vi "Set_Tunnel_Speed.vi"(3 "Mode":T1, 4 "Rig Name (default Empty)":string, 5 "Tunnel Velocity m/s":dbl min=0.0 max=50.0 format="%#.3f") -> (0 "Error String":string, 2 "Max allowable Tunnel Velocity":dbl)   [LabVIEW 2022 SP3]
doc: "This is an example of using features of the VI Server as a client. It shows how you might browse from one or more applications that may be exporting data from one or more data stations. \n\nThe example shows how to query a server for its list of exported VIs, how to get references to the VIs, and how call them with the Call By Reference function."
uses:
  Sub VIs/ADAM Controls/Tunnel_speed_mode.ctl
  Sub VIs/ADAM Controls/Channel_State.ctl
  Anemometry/Anemometry Sub Vis/File/Setup_Filetype.ctl
  Sub VIs/ADAM Controls/Update_scan_value.ctl
  Anemometry/Anemometry Sub Vis/Controls/Global_mode.ctl
  Sub VIs/ADAM Controls/Ch_description_ADAM.ctl
  Sub VIs/ADAM Controls/Module_type_ADAM.ctl
  Sub VIs/ADAM Controls/Function_ADAM.ctl
  Sub VIs/ADAM Controls/Calib_type_ADAM.ctl
  Sub VIs/ADAM Controls/Address.ctl
  Anemometry/Anemometry Sub Vis/Globals/Preference_global.vi
  Anemometry/Anemometry Sub Vis/Globals/Constants_global.vi
  <vilib>/Analysis/NI_AALPro.lvlib
panel:
  out "Motor Enable On?":bool
  out "i count":i32
  out "Settling Time (s)":dbl
  in  "Set EnFlo Tun Speed":refnum<vi>
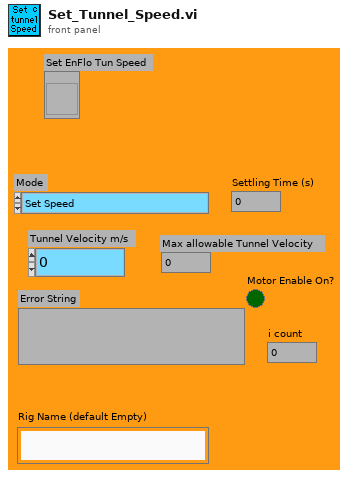
[diagram p1: front panel]
types:
  T1 = typedef "Tunnel_speed_mode.ctl" = enum16{"Set Speed", "Set Speed then wait", "Is tunnel speed allowable?"}
  T2 = typedef "Channel_State.ctl" = enum16{"On", "Off", "Always On", "Always Off"}
  T3 = enum16{"On", "Off", "Always On", "Always Off", "Delete"}
  T4 = typedef "Setup_Filetype.ctl" = enum16{"Measurement Setups", "Calibration Setups", "General", "Results File Plotter Setups", "Speed Calib Tweaks"}
  T5 = typedef "Calib_type_ADAM.ctl" = string
  T6 = typedef "Module_type_ADAM.ctl" = string
  T7 = typedef "Ch_description_ADAM.ctl" = cluster{"Ch Name":string, "Type":T6, "Function":T8, "Ch State":T2, "Calibration type":T5, "A":dbl, "B":dbl, "C":dbl, "D":dbl, "Comments":string, "Address":T9, "String":string, "Duty":u16}
  T8 = typedef "Function_ADAM.ctl" = enum16{"Analogue Input", "Digital Input", "Event counter", "Event rate", "Analogue Output", "Digital Output", "Relay Output"}
  T9 = typedef "Address.ctl" = cluster{"Main":i32, "Ch.":i32, "Sub":i32, "Port Name":string}
  T10 = typedef "Global_mode.ctl" = enum16{"Read Global", "Load Global From File", "Write Global to File"}
  T11 = typedef "Update_scan_value.ctl" = cluster{"Channel Name":string, "New Value":dbl, "!Auto_Off":bool}
  T12 = typedef "Server_Comms.ctl" = enum16{"Do Not Link To Server", "Server Link Healthy"}
  T13 = cluster{"second":i32, "minute":i32, "hour":i32, "day of month":i32, "month":i32, "year":i32, "day of week":i32, "day of year":i32, "is DST":i32}
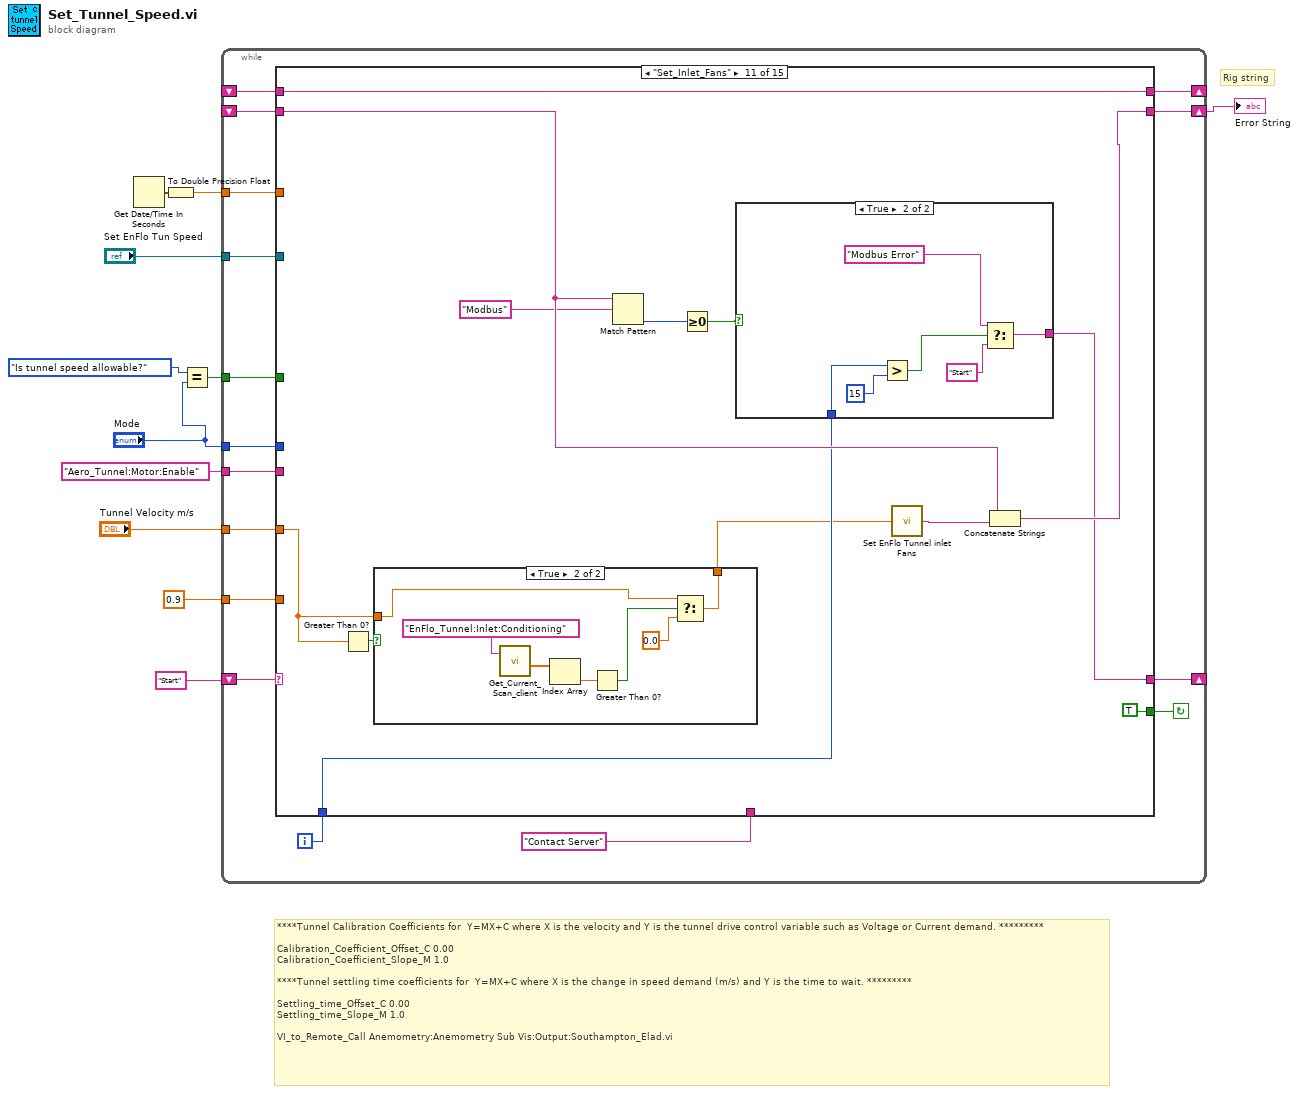
[diagram p0: block diagram]
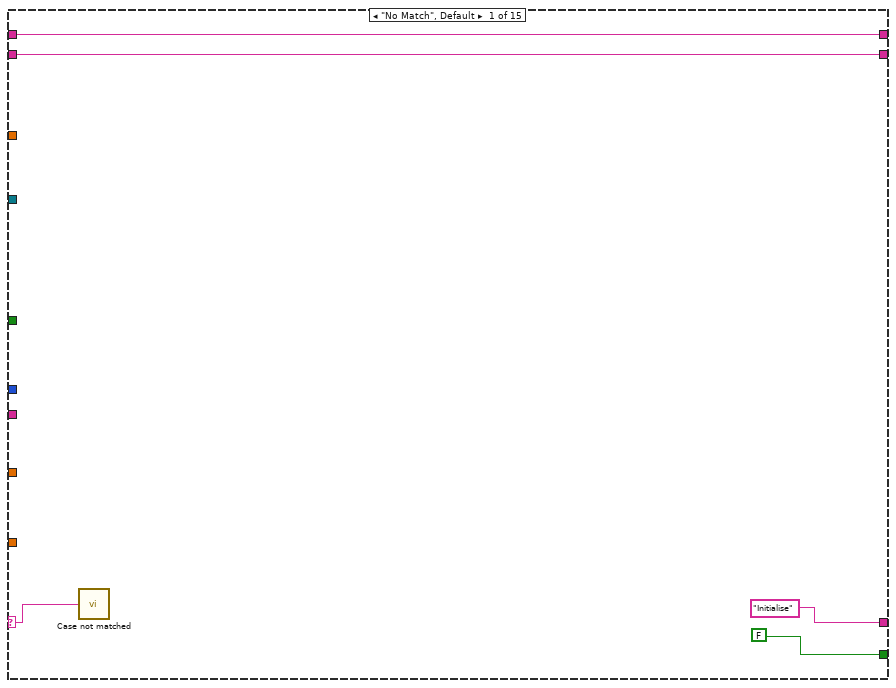
[diagram p2: hidden frame]
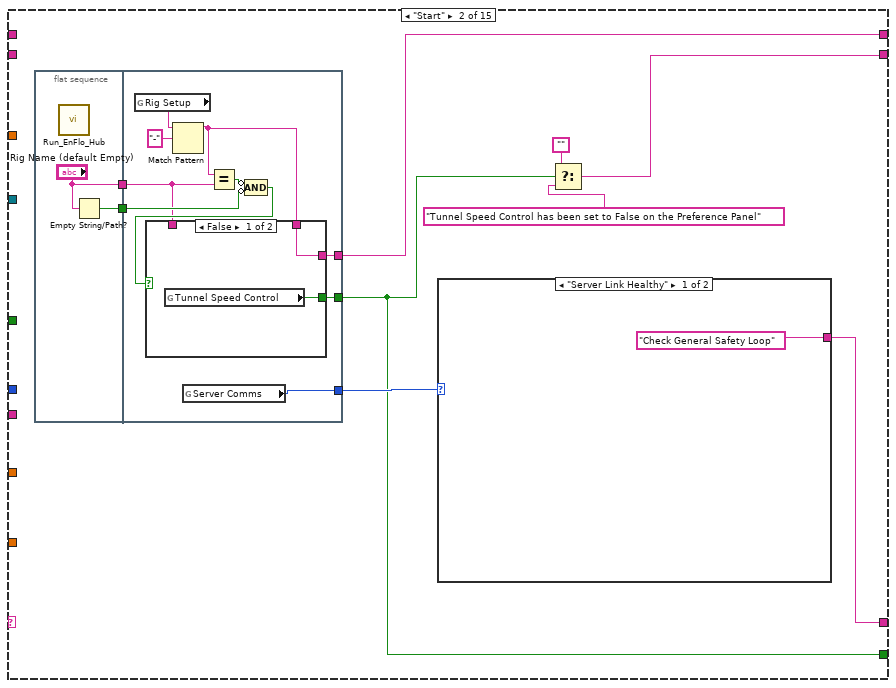
[diagram p3: hidden frame]
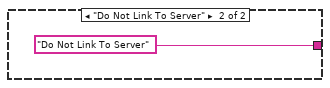
[diagram p4: hidden frame]
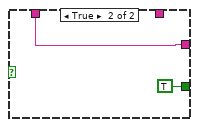
[diagram p5: hidden frame]
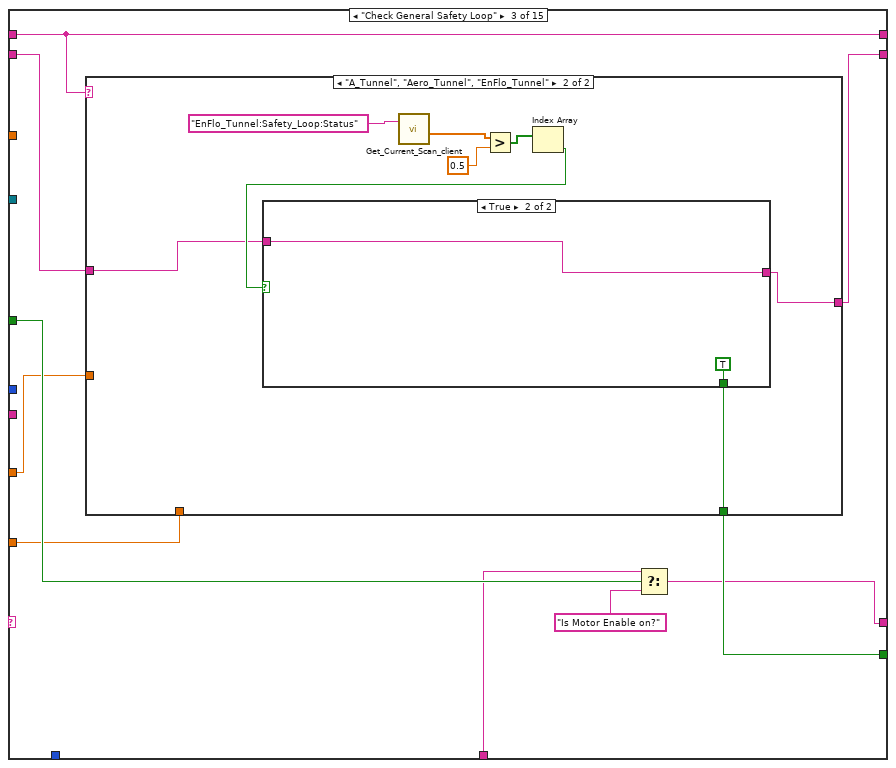
[diagram p6: hidden frame]
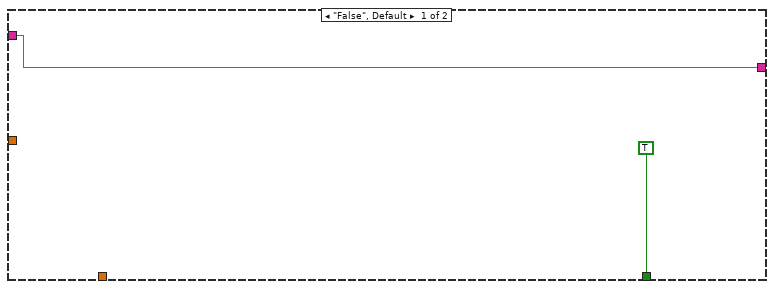
[diagram p7: hidden frame]
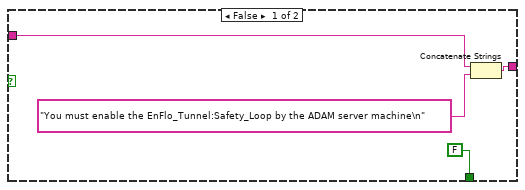
[diagram p8: hidden frame]
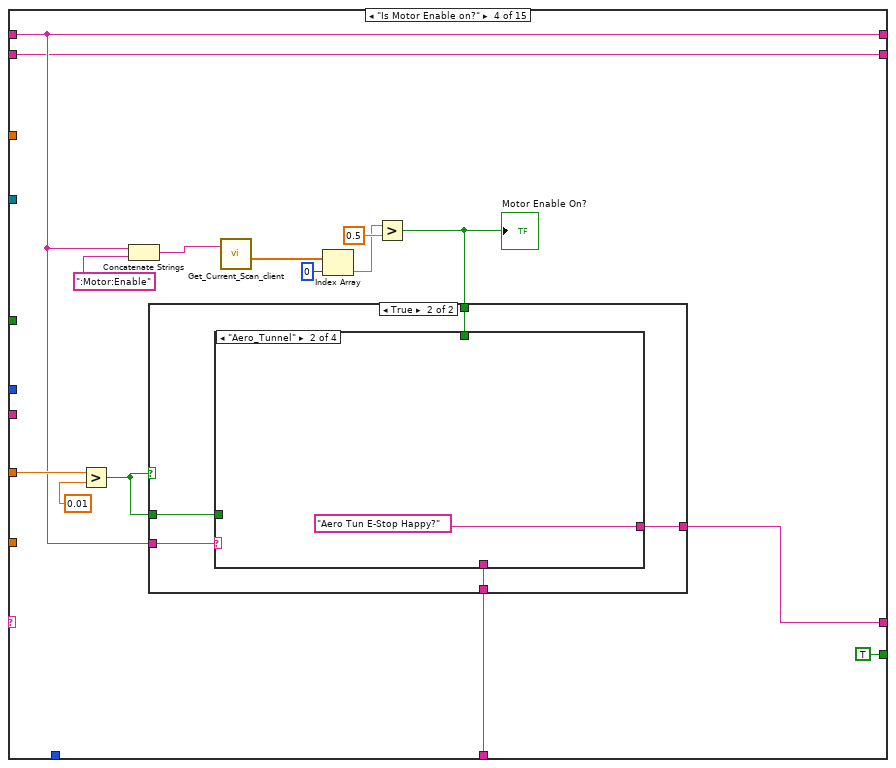
[diagram p9: hidden frame]
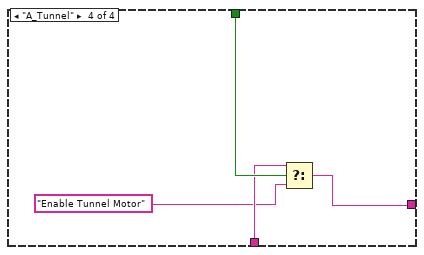
[diagram p13: hidden frame]
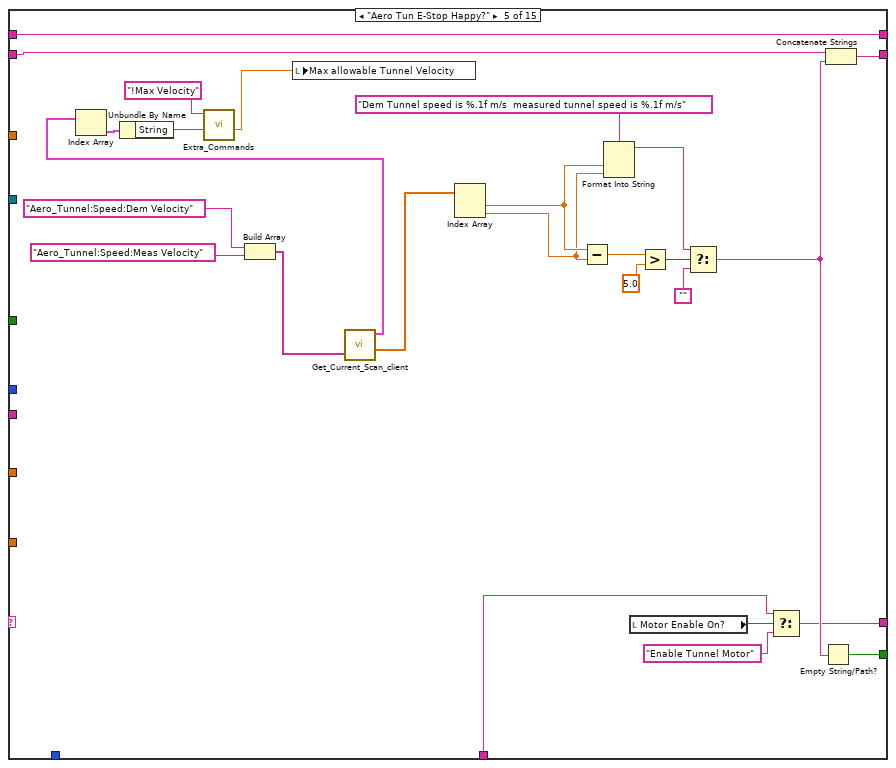
[diagram p14: hidden frame]
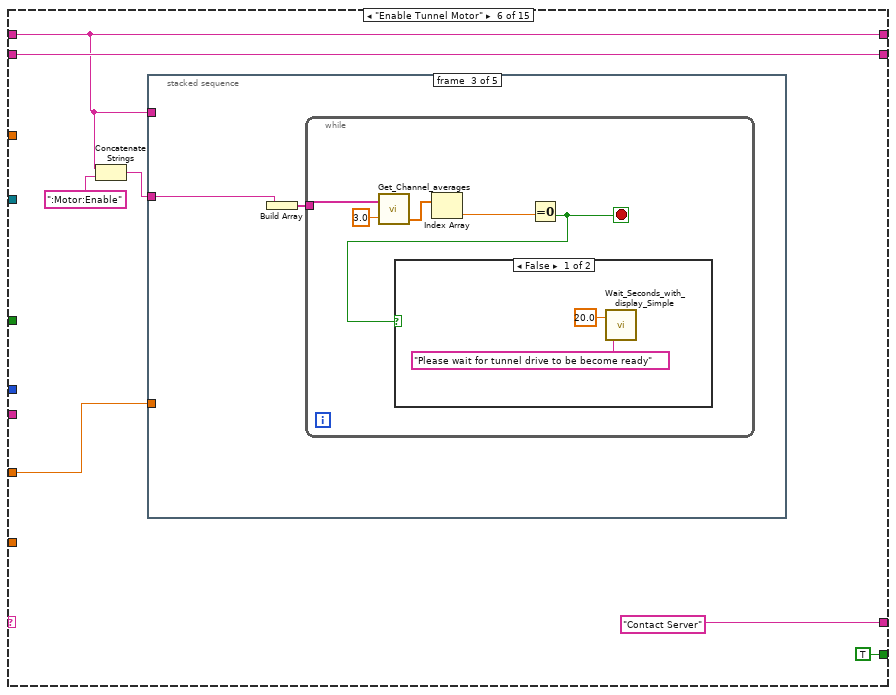
[diagram p15: hidden frame]
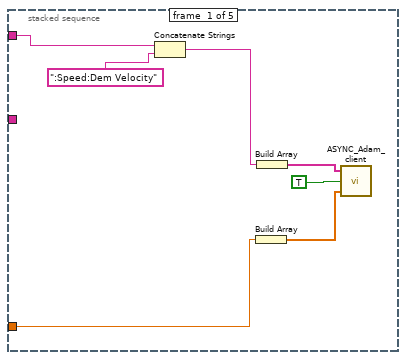
[diagram p16: hidden frame]
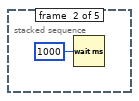
[diagram p17: hidden frame]
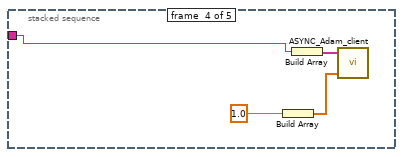
[diagram p19: hidden frame]
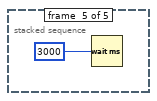
[diagram p20: hidden frame]
diagram:
  # "Rig string"
  # "****Tunnel Calibration Coefficients for  Y=MX+C where X is the velocity and Y is the tunnel drive control variable such as Voltage or Current demand. *********\n\nCalibration_Coefficient_Offset_C\t0.00\nCalibration_Coefficient_Slope_M\t1.0\n\n****Tunnel settling time coefficients for  Y=MX+C where X is the change in speed demand (m/s) and Y is the time to wait. *********\n\nSettling_time_Offset_C\t0.00\nSettling_time_Slope_M\t1.0\n\nVI_to_Remote_Call\tAnemometry:Anemometry Sub Vis:Output:Southampton_Elad.vi"
  n1 = Get Date/Time In Seconds() -> (seconds since 1Jan1904=w7:timestamp)
  n2 = To Double Precision Float(number=w7) -> (double precision float=w6:dbl)
  n3 = Equal?(x=Tunnel_speed_mode."Is tunnel speed allowable?" ("Mode"), y="Mode") -> (x = y?=w2:bool)
  n4 = while {
    shift-left: "Start" -> [w26]
    shift-right: [w27] -> _
    shift-right: [w25] -> w10
    shift-left: _ -> [w24]
    tunnel: "Mode" -> [w23]
    tunnel: "Tunnel Velocity m/s" -> [w22]
    shift-right: [w21] -> _
    shift-left: _ -> [w20]
    tunnel: "Set EnFlo Tun Speed" -> [w18]
    tunnel: w6 -> [w17]
    tunnel: "Aero_Tunnel:Motor:Enable" -> [w16]
    tunnel: 0.9 ("y") -> [w15]
    tunnel: w2 -> [w14]
    i -> [w13]
    stop <- w19 continue-if-true
    n5 = case shown="\"Set_Inlet_Fans\"" w26 {
      selector: w26 -> [w28 _ _ _ _ _ _ _ _ _ _ _ _ _ _]
      tunnel: [FALSE w40 w69 TRUE ("Tunnel Speed Control") w126 TRUE ("Tunnel Speed Control") w173 TRUE ("Tunnel Speed Control") w240 w357 TRUE ("Tunnel Speed Control") w427 w475 FALSE ("Tunnel Speed Control") FALSE] -> w19
      tunnel: ["Initialise" w36 w62 w92 w114 "Contact Server" ("f") w169 "Contact Server" ("f") w239 "Aero Tunnel Steady?" ("f") w401 w426 "Start" "End" ("f") "End"] -> w27
      tunnel: [w30 w38 w67 w89 w132 w146 w187 w215 w235 w381 w406 w430 w478 w499 w505] -> w25
      tunnel: w24 -> [w30 _ w68 w89 w133 w146 w189 w215 w236 w381 w405 w430 w478 w499 w503]
      tunnel: w23 -> [_ _ _ _ _ _ w186 _ w238 _ _ _ _ w492 w507]
      tunnel: w22 -> [_ _ w61 w94 _ w143 _ w222 w233 w360 w397 _ _ _ w506]
      tunnel: [w29 w35 w66 w93 w139 w140 w192 w211 w241 w382 w409 w431 w479 w500 w504] -> w21
      tunnel: w20 -> [w29 _ w66 w93 w139 w140 w192 w211 w241 w382 w409 w431 w479 w500 w504]
      tunnel: w18 -> [_ _ _ _ _ _ _ _ w242 _ _ _ _ _ _]
      tunnel: w17 -> [_ _ _ _ _ _ _ _ w234 _ _ _ _ _ _]
      tunnel: w16 -> [_ _ _ _ _ _ _ _ _ w344 _ _ _ _ _]
      tunnel: w15 -> [_ _ w60 _ _ _ _ _ w232 _ _ _ _ _ _]
      tunnel: w14 -> [_ _ w65 _ _ _ _ w214 w231 _ _ _ _ _ _]
      tunnel: w13 -> [_ _ _ _ _ _ _ _ _ w362 w400 w429 w477 _ _]
      tunnel: "Contact Server" ("f") -> [_ _ w64 w86 w115 _ _ _ _ _ _ _ _ _ _]
      frame "No Match", Default {
        n6 = call "Case not matched.vi"("Case Name not Matched"=w28) -> ()
      }
      frame "Start" {
        n7 = flat-sequence {
          tunnel: ["Rig Name (default Empty)"] -> w34
          tunnel: [w44] -> w33
          tunnel: [w55] -> w41
          tunnel: [w49] -> w40
          tunnel: [w48] -> w35
          tunnel: w34 -> [w46]
          tunnel: w33 -> [w51]
          frame #0 {
            n8 = call "Run_EnFlo_Hub.vi"() -> ()  [unwired: 1 in, 7 out]
            n9 = Empty String/Path?(string/path="Rig Name (default Empty)") -> (empty?=w44:bool)
          }
          frame #1 {
            n10 = global read "Preference_global.vi" "Rig Setup"() -> (w54:string)
            n11 = Match Pattern(string=w54, regular expression="-") -> (before substring=w47:string)  [unwired: 4 out]
            n12 = global read "Preference_global.vi" "Server Comms"() -> (w55:T12)
            n13 = Equal?(x=w47, y=w46) -> (x = y?=w52:bool)
            n14 = Compound Arithmetic op=AND(invert w52, invert w51) -> (w50:bool)
            n15 = case shown="False" w50 {
              tunnel: [w57 TRUE ("Tunnel Speed Control")] -> w49
              tunnel: [w56 w58] -> w48
              tunnel: w47 -> [w56 _]
              tunnel: w46 -> [_ w58]
              frame False {
                n16 = global read "Preference_global.vi" "Tunnel Speed Control"() -> (w57:bool)
              }
              frame True {
              }
            }
          }
        }
        n17 = case shown="\"Server Link Healthy\"" w41 {
          tunnel: ["Check General Safety Loop" "Do Not Link To Server"] -> w36
          frame "Server Link Healthy" {
          }
          frame "Do Not Link To Server" {
          }
        }
        n18 = Select(t="", s=w40, f="Tunnel Speed Control has been set to False on the Preference Panel" ("Error String")) -> (s? t:f=w38:string)
      }
      frame "Check General Safety Loop" {
        n19 = case shown="\"A_Tunnel\", \"Aero_Tunnel\", \"EnFlo_Tunnel\"" w66 {
          tunnel: w68 -> [w70 w74]
          tunnel: [w70 w73] -> w67
          tunnel: [TRUE ("Tunnel Speed Control") w72] -> w69
          tunnel: w61 -> [_ _]
          tunnel: w60 -> [_ _]
          frame "False", Default {
          }
          frame "A_Tunnel", "Aero_Tunnel", "EnFlo_Tunnel" {
            n20 = call "Get_Current_Scan_client.vi"("singleChannel"="EnFlo_Tunnel:Safety_Loop:Status") -> ("Numerical Values"=w77:dbl[])  [unwired: 1 in, 3 out]
            n21 = Greater?(x=w77, y=0.5) -> (0:w78:bool[])
            n22 = Index Array(array=w78) -> (element=w75:bool)  [unwired: 1 in]
            n23 = case shown="True" w75 {
              tunnel: [w83 w84] -> w73
              tunnel: w74 -> [w81 w84]
              tunnel: [FALSE ("Tunnel Speed Control") TRUE ("Tunnel Speed Control")] -> w72
              frame False {
                n24 = Concatenate Strings(w81, "You must enable the EnFlo_Tunnel:Safety_Loop by the ADAM server machine\n") -> (w83:string)
              }
              frame True {
              }
            }
          }
        }
        n25 = Select(t=w64, s=w65, f="Is Motor Enable on?") -> (s? t:f=w62:string)
      }
      frame "Is Motor Enable on?" {
        n26 = Greater?(x=w94, y=0.01) -> (0:w88:bool)
        n27 = Concatenate Strings(w93, ":Motor:Enable" ("string")) -> (w91:string)
        n28 = call "Get_Current_Scan_client.vi"("singleChannel"=w91) -> ("Numerical Values"=w96:dbl[])  [unwired: 1 in, 3 out]
        n29 = Index Array(array=w96, index=0) -> (element=w98:dbl)
        n30 = Greater?(x=w98, y=0.5) -> (0:w90:bool)
        "Motor Enable On?" <- w90
        n31 = case shown="True" w88 {
          tunnel: w93 -> [_ w106]
          tunnel: w86 -> [w101 w105]
          tunnel: [w101 w104] -> w92
          tunnel: w90 -> [_ w103]
          tunnel: w88 -> [_ w102]
          frame False {
          }
          frame True {
            n32 = case shown="\"Aero_Tunnel\"" w106 {
              selector: w106 -> [_ _ w109 _]
              tunnel: [w107 "Aero Tun E-Stop Happy?" ("f") w109 w110] -> w104
              tunnel: w105 -> [w107 _ _ w112]
              tunnel: w103 -> [_ _ _ w113]
              tunnel: w102 -> [_ _ _ _]
              frame Default {
              }
              frame "Aero_Tunnel" {
              }
              frame "EnFlo_Tunnel" {
              }
              frame "A_Tunnel" {
                n33 = Select(t=w112, s=w113, f="Enable Tunnel Motor") -> (s? t:f=w110:string)
              }
            }
          }
        }
      }
      frame "Aero Tun E-Stop Happy?" {
        n34 = Build Array("Aero_Tunnel:Speed:Dem Velocity", "Aero_Tunnel:Speed:Meas Velocity") -> (w136:string[])
        n35 = call "Get_Current_Scan_client.vi"("multipleChannels"=w136) -> ("Ch Description Array"=w123:T7[], "Numerical Values"=w119:dbl[])  [unwired: 1 in, 2 out]
        n36 = Index Array(array=w123) -> (element=w122:T7)  [unwired: 1 in]
        n37 = Unbundle By Name(w122) -> ("String"=w124:string)
        n38 = call "Extra_Commands.vi"("String to Search"=w124, "Command"="!Max Velocity") -> ("Numeric Value"=w121:dbl)  [unwired: 1 in, 4 out]
        n39 = local write "Max allowable Tunnel Velocity"(w121) -> ()
        n40 = Index Array(array=w119) -> (element #1=w131:dbl, element #2=w118:dbl)  [unwired: 2 in]
        n41 = Subtract(x=w131, y=w118) -> (x-y=w135:dbl)
        n42 = Format Into String(format string="Dem Tunnel speed is %.1f m/s  measured tunnel speed is %.1f m/s", w131, w118) -> (resulting string=w129:string)  [unwired: 2 in, 1 out]
        n43 = local read "Motor Enable On?"() -> (w117:bool)
        n44 = Greater?(x=w135, y=5.0) -> (0:w128:bool)
        n45 = Select(t=w129, s=w128, f="") -> (s? t:f=w120:string)
        n46 = Select(t=w115, s=w117, f="Enable Tunnel Motor") -> (s? t:f=w114:string)
        n47 = Empty String/Path?(string/path=w120) -> (empty?=w126:bool)
        n48 = Concatenate Strings(w133, w120) -> (w132:string)
      }
      frame "Enable Tunnel Motor" {
        n49 = Concatenate Strings(w140, ":Motor:Enable" ("string")) -> (w141:string)
        n50 = stacked-sequence {
          tunnel: w141 -> [_ _ w156 w164 _]
          tunnel: w143 -> [w151 _ _ _ _]
          tunnel: w140 -> [w149 _ _ _ _]
          frame #0 {
            n51 = Concatenate Strings(w149, ":Speed:Dem Velocity" ("string")) -> (w147:string)
            n52 = Build Array(w151) -> (w150:dbl[])
            n53 = Build Array(w147) -> (w153:string[])
            n54 = call "ASYNC_Adam_client.vi"("Values"=w150, "Check Value is in the scan table?"=TRUE, "Channel Names"=w153) -> ()  [unwired: 2 out]
          }
          frame #1 {
            n55 = Wait (ms)(milliseconds to wait=u32 1000) -> ()  [unwired: 1 out]
          }
          frame #2 {
            n56 = Build Array(w156) -> (w155:string[])
            n57 = while {
              tunnel: w155 -> [w161]
              stop <- w157 stop-if-true
              n58 = call "Get_Channel_averages.vi"("Desired Ch Names"=w161, "Averaging time (mins)"=3.0) -> ("number"=w159:dbl[])  [unwired: 1 in, 2 out]
              n59 = Index Array(array=w159) -> (element=w158:dbl)  [unwired: 1 in]
              n60 = Equal To 0?(x=w158) -> (x = 0?=w157:bool)
              n61 = case shown="False" w157 {
                frame False {
                  n62 = call "Wait_Seconds_with_display_Simple.vi"("Message"="Please wait for tunnel drive to be become ready", "Seconds to wait"=20.0) -> ()  [unwired: 1 in, 1 out]
                }
                frame True {
                }
              }
            }
          }
          frame #3 {
            n63 = Build Array(1.0 ("y")) -> (w166:dbl[])
            n64 = Build Array(w164) -> (w165:string[])
            n65 = call "ASYNC_Adam_client.vi"("Values"=w166, "Channel Names"=w165) -> ()  [unwired: 1 in, 2 out]
          }
          frame #4 {
            n66 = Wait (ms)(milliseconds to wait=u32 3000 ("millisecond timer value")) -> ()  [unwired: 1 out]
          }
        }
      }
      frame "EnFlo_Tunnel" {
        w175 = "EnFlo_Tunnel:Drive:In Standby"
        w182 = "EnFlo_Tunnel:Bus Bar + Heaters:Enable"
        n67 = Build Array(w182, w175, "EnFlo_Tunnel:Emergency_Stop:Happy") -> (w190:string[])
        n68 = call "Get_Current_Scan_client.vi"("multipleChannels"=w190) -> ("Ch Description Array"=w181:T7[], "Numerical Values"=w185:dbl[])  [unwired: 1 in, 2 out]
        n69 = Greater?(x=w185, y=0.5) -> (0:w184:bool[])
        n70 = Index Array(array=w184) -> (element #1=w183:bool, element #3=w173:bool)  [unwired: 3 in, 1 out]
        n71 = case shown="True" w173 {
          tunnel: w182 -> [_ w200]
          tunnel: ["The EnFlo_Tunnel Emergency Stop button has been pressed. You need to reset it before running." w199] -> w188
          tunnel: w186 -> [_ w198]
          tunnel: w183 -> [_ w197]
          frame False {
          }
          frame True {
            n72 = case shown="False" w197 {
              tunnel: w200 -> [w203 _]
              tunnel: ["" ""] -> w199
              tunnel: w198 -> [w201 _]
              frame False {
                n73 = case shown="Default" w201 {
                  tunnel: w203 -> [_ w207]
                  frame "Is tunnel speed allowable?" {
                  }
                  frame Default {
                    n74 = Build Array(w207, "EnFlo_Tunnel:Shutting:Down") -> (w206:string[])
                    n75 = Build Array(1.0 ("element"), 0.0 ("element")) -> (w209:dbl[])
                    n76 = call "ASYNC_Adam_client.vi"("Values"=w209, "Channel Names"=w206) -> ()  [unwired: 1 in, 2 out]
                  }
                }
              }
              frame True {
              }
            }
          }
        }
        n77 = Index Array(array=w181, index=1) -> (element=w179:T7)
        n78 = Unbundle By Name(w179) -> ("Ch State"=w178:T2)
        n79 = local read "Motor Enable On?"() -> (w172:bool)
        n80 = Equal?(x=w178, y=Channel_State."Off") -> (x = y?=w176:bool)
        n81 = Concatenate Strings(w189, w188) -> (w187:string)
        n82 = case shown="True" w176 {
          tunnel: w175 -> [_ w195]
          frame False {
          }
          frame True {
            n83 = Build Array(w195) -> (w194:string[])
            n84 = call "Cntrl_Ch_Status_low.vi"("Mode"=T3."On", "Channel names"=w194) -> ()  [unwired: 1 out]
          }
        }
        n85 = Select(t="Contact Server" ("f"), s=w172, f="Enable EnFlo Tunnel Motor") -> (s? t:f=w169:string)
      }
      frame "Enable EnFlo Tunnel Motor" {
        n86 = Greater?(x=w222, y=0.15) -> (0:w220:bool)
        n87 = Concatenate Strings(w211, ":Motor:Enable" ("string")) -> (w212:string)
        n88 = Build Array(w212) -> (w217:string[])
        n89 = Compound Arithmetic op=AND(w220, invert w214) -> (w218:bool)
        n90 = case shown="True" w218 {
          tunnel: w217 -> [_ w223]
          frame False {
          }
          frame True {
            n91 = stacked-sequence {
              tunnel: w223 -> [w227 _]
              frame #0 {
                n92 = Build Array(1.0 ("y")) -> (w229:dbl[])
                n93 = Build Array("EnFlo_Tunnel:Drive:In Standby") -> (w226:string[])
                n94 = call "ASYNC_Adam_client.vi"("Values"=w229, "Channel Names"=w227) -> ()  [unwired: 1 in, 2 out]
                n95 = call "Cntrl_Ch_Status_low.vi"("Mode"=T3."On", "Channel names"=w226) -> ()  [unwired: 1 out]
              }
              frame #1 {
                n96 = Wait (ms)(milliseconds to wait=u32 3000 ("millisecond timer value")) -> ()  [unwired: 1 out]
              }
            }
          }
        }
      }
      frame "Contact Server" {
        n97 = while {
          tunnel: w238 -> [w278]
          tunnel: w233 -> [w279]
          shift-left: _ -> [w275]
          shift-right: [w282] -> _
          tunnel: [w277] -> w237
          tunnel: w241 -> [w276]
          tunnel: w242 -> [w274]
          tunnel: w234 -> [w273]
          i -> [w281]
          stop <- w280 continue-if-true
          n98 = stacked-sequence {
            seq-local: [_ w291 _ _] -> [_ _ w299 _]
            seq-local: [_ w290 _ _] -> [_ _ w297 _]
            seq-local: [_ _ w293 _] -> [_ _ _ w325]
            tunnel: w275 -> [_ w292 _ _]
            tunnel: [_ _ w300 _] -> w282
            tunnel: w281 -> [_ _ _ w326]
            tunnel: [_ _ _ w324] -> w280
            tunnel: w279 -> [_ w288 _ _]
            tunnel: w278 -> [_ w284 _ _]
            tunnel: [_ w286 _ _] -> w277
            tunnel: w276 -> [_ w285 _ _]
            tunnel: w274 -> [_ _ w296 _]
            tunnel: w273 -> [_ _ w294 _]
            frame #0 {
            }
            frame #1 {
              n99 = call "Full_Client_Name.vi"() -> ("Client Name"=w289:string)
              n100 = call-by-ref "?"(reference=w292, "Tunnel Velocity m/s"=w288, "Rig Name"=w285, "Mode"=w284, "Client Name"=w289) -> (reference out=w291:refnum<vi>, error out=w290:errorcluster, "Error String"=w286:string, "Settling Time (s)"=→"Settling Time (s)":dbl, "Max allowable Tunnel Velocity"=→"Max allowable Tunnel Velocity":dbl)  [unwired: 1 in, 1 out]
            }
            frame #2 {
              n101 = Unbundle By Name(w297) -> ("status"=w298:bool)
              n102 = case shown="False" w298 {
                selector: w298 -> [w301 _]
                tunnel: [w302 w309] -> w300
                tunnel: w299 -> [w302 _]
                tunnel: [w303 w308] -> w295
                tunnel: w297 -> [w303 _]
                tunnel: w296 -> [_ w307]
                tunnel: [w301 w305] -> w293
                frame False {
                }
                frame True {
                  n103 = call "Start_Client_Coms.vi"("VI name to run on server"="Set_Tunnel_Speed_server.vi") -> ("LabVIEW application reference"=w311:refnum<vi>, "Checked VI name"=w312:path, "Local Call"=w310:bool, "Error cluster"=w304:errorcluster)  [unwired: 1 in]
                  n104 = case shown="False" w310 {
                    tunnel: [w318 w323] -> w309
                    tunnel: w307 -> [w316 w322]
                    tunnel: w312 -> [w315 w321]
                    tunnel: w311 -> [w314 _]
                    tunnel: [w317 w320] -> w308
                    frame False {
                      n105 = Strip Path(path=w315) -> (name=w319:string)  [unwired: 1 out]
                      n106 = Open VI Reference(type specifier VI Refnum (for type only)=w316, application reference (local)=w314, vi path=w319) -> (vi reference=w318:refnum<vi>, error out=w317:errorcluster)  [unwired: 1 in, 2 out]
                    }
                    frame True {
                      n107 = Open VI Reference(type specifier VI Refnum (for type only)=w322, vi path=w321) -> (vi reference=w323:refnum<vi>, error out=w320:errorcluster)  [unwired: 1 in, 3 out]
                    }
                  }
                  n108 = Unbundle By Name(w304) -> ("status"=w306:bool)
                  n109 = Not(x=w306) -> (.not. x?=w305:bool)
                }
              }
              n110 = call "Delay Error Message.vi"("error in (no error)"=w295, "Seconds since 1904"=w294) -> ()  [unwired: 2 in]
            }
            frame #3 {
              n111 = Less?(x=w326, y=30) -> (x < y?=w328:bool)
              n112 = And(x=w328, y=w325) -> (x .and. y?=w324:bool)
            }
          }
        }
        n113 = case shown="\"EnFlo_Tunnel\"" w241 {
          tunnel: [TRUE w248 w268] -> w240
          tunnel: ["Tunnel Speed Settling" ("f") "Aero Tunnel Steady?" ("f") "Set_Inlet_Fans" ("f")] -> w239
          tunnel: w238 -> [_ w249 w270]
          tunnel: w233 -> [_ w247 _]
          tunnel: w232 -> [_ w246 _]
          tunnel: w231 -> [_ w245 _]
          frame "No Match", Default {
          }
          frame "Aero_Tunnel" {
            n114 = case shown="False" w245 {
              tunnel: w247 -> [w260 _]
              tunnel: w246 -> [w259 _]
              frame False {
                w252 = "Aero_Tunnel:Motor:Engaged"
                n115 = Greater?(x=w260, y=w259) -> (0:w253:bool)
                n116 = call "Get_Current_Scan_client.vi"("singleChannel"=w252) -> ("Numerical Values"=w258:dbl[])  [unwired: 1 in, 3 out]
                n117 = Index Array(array=w258) -> (element=w257:dbl)  [unwired: 1 in]
                n118 = Greater?(x=w257, y=0.5) -> (0:w255:bool)
                n119 = Equal?(x=w255, y=w253) -> (x = y?=w254:bool)
                n120 = case shown="False" w254 {
                  tunnel: w252 -> [w266 _]
                  tunnel: w253 -> [w264 _]
                  frame False {
                    n121 = Select(t=1.0, s=w264, f=0.0) -> (s? t:f=w261:dbl)
                    n122 = Build Array(w266) -> (w265:string[])
                    n123 = Build Array(w261) -> (w267:dbl[])
                    n124 = call "ASYNC_Adam_client.vi"("Values"=w267, "Channel Names"=w265) -> ()  [unwired: 1 in, 2 out]
                  }
                  frame True {
                  }
                }
              }
              frame True {
              }
            }
            n125 = Equal?(x=Tunnel_speed_mode."Set Speed then wait" ("Mode"), y=w249) -> (x = y?=w248:bool)
          }
          frame "EnFlo_Tunnel" {
            n126 = Equal?(x=Tunnel_speed_mode."Is tunnel speed allowable?" ("Mode"), y=w270) -> (x = y?=w269:bool)
            n127 = Not(x=w269) -> (.not. x?=w268:bool)
          }
        }
        n128 = Concatenate Strings(w236, w237) -> (w235:string)
      }
      frame "Aero Tunnel Steady?" {
        w351 = string[] ["Aero_Tunnel:Speed:Meas Velocity", "Aero_Tunnel:Speed:Dem Velocity"] ("ADAM Ch Names")
        n129 = Index Array(array=w351, index=1) -> (element=w349:string)
        n130 = Build Array(w349, w344) -> (w348:string[])
        n131 = call "Get_Ch_Time_Trace.vi"("Desired Ch Names"=w348, "History Length (mins)"=4.0) -> ("Output array"=w342:dbl[][])  [unwired: 2 out]
        n132 = Index Array(array=w342, index (row)=1) -> (element=w340:dbl[])  [unwired: 1 in]
        n133 = Equal To 0?(x=w340) -> (x = 0?=w341:bool[])
        n134 = Index Array(array=w342, index (row)=0) -> (element=w346:dbl[])  [unwired: 1 in]
        n135 = call "Get_Ch_Time_Trace.vi"("Desired Ch Names"=w351, "History Length (mins)"=0.3) -> ("Centre Times"=w335:dbl[], "Output array"=w377:dbl[][])  [unwired: 1 out]
        n136 = And Array Elements(Boolean array=w341) -> (logical AND=w338:bool)
        n137 = Equal To 0?(x=w346) -> (x = 0?=w345:bool[])
        n138 = And Array Elements(Boolean array=w345) -> (logical AND=w339:bool)
        n139 = Greater?(x=w360, y=4.0) -> (0:w358:bool)
        n140 = Less?(x=w362, y=18) -> (x < y?=w355:bool)
        n141 = Or(x=w339, y=w338) -> (x .or. y?=w337:bool)
        n142 = Index Array(array=w377, index (row)=0) -> (element=w336:dbl[])  [unwired: 1 in]
        n143 = Index Array(array=w377, index (row)=1) -> (element=w369:dbl[])  [unwired: 1 in]
        n144 = call "Mean_fr_NaN_data.vi"("Data"=w369) -> ("Mean value"=w368:dbl)  [unwired: 1 out]
        n145 = call <vilib>:"Linear Fit.vi"("Y"=w336, "X"=w335) -> ("Best Linear Fit"=w333:dbl[])  [unwired: 9 in, 4 out]
        n146 = Subtract(x=w368, y=w360) -> (x-y=w374:dbl)
        n147 = Array Size(array=w333) -> (size(s)=w332:i32)
        n148 = In Range and Coerce(upper limit=0.01, x=w374, lower limit=-0.01) -> (In Range?=w373:bool)  [unwired: 1 out]
        n149 = Decrement(x=w332) -> (x-1=w331:i32)
        n150 = Not A Number/Path/Refnum?(number/path/refnum=w368) -> (NaN/Path/Refnum?=w370:bool)
        n151 = Not A Number/Path/Refnum?(number/path/refnum=w336) -> (NaN/Path/Refnum?=w354:bool[])
        n152 = Not(x=w373) -> (.not. x?=w372:bool)
        n153 = And Array Elements(Boolean array=w354) -> (logical AND=w353:bool)
        n154 = Index Array(array=w333, index #1=0 ("index"), index #2=w331) -> (element #1=w330:dbl, element #2=w329:dbl)
        n155 = Subtract(x=w330, y=w329) -> (x-y=w365:dbl)
        n156 = In Range and Coerce(upper limit=0.2, x=w365, lower limit=-0.2) -> (In Range?=w364:bool)  [unwired: 1 out]
        n157 = Not(x=w364) -> (.not. x?=w363:bool)
        n158 = Or(x=w363, y=w372) -> (x .or. y?=w371:bool)
        n159 = Compound Arithmetic op=AND(invert w353, w371, invert w370) -> (w356:bool)
        n160 = case shown="True" w337 {
          tunnel: w358 -> [w387 _]
          tunnel: [w386 FALSE] -> w357
          tunnel: w356 -> [w385 _]
          tunnel: w355 -> [w384 _]
          frame False {
            n161 = case shown="False" w387 {
              tunnel: [w389 w393] -> w386
              tunnel: w385 -> [w390 w393]
              tunnel: w384 -> [w388 _]
              frame False {
                n162 = case shown="True" w390 {
                  selector: w390 -> [w391 _]
                  tunnel: [w391 w392] -> w389
                  tunnel: w388 -> [_ w392]
                  frame False {
                  }
                  frame True {
                  }
                }
              }
              frame True {
              }
            }
          }
          frame True {
          }
        }
        n163 = case shown="True" w357 {
          frame False {
          }
          frame True {
            n164 = call "Wait_Seconds_with_display.vi"("Message"="Tunnel speed settling", "Seconds to wait"=4.0) -> ()  [unwired: 2 out]
          }
        }
        "i count" <- w362
      }
      frame "Set_Inlet_Fans" {
        n165 = Greater Than 0?(x=w397) -> (x > 0?=w399:bool)
        n166 = case shown="True" w399 {
          tunnel: [w410 w411] -> w398
          tunnel: w397 -> [w410 w413]
          frame False {
          }
          frame True {
            n167 = call "Get_Current_Scan_client.vi"("singleChannel"="EnFlo_Tunnel:Inlet:Conditioning") -> ("Numerical Values"=w416:dbl[])  [unwired: 1 in, 3 out]
            n168 = Index Array(array=w416) -> (element=w415:dbl)  [unwired: 1 in]
            n169 = Greater Than 0?(x=w415) -> (x > 0?=w414:bool)
            n170 = Select(t=w413, s=w414, f=0.0) -> (s? t:f=w411:dbl)
          }
        }
        n171 = Match Pattern(string=w405, regular expression="Modbus") -> (offset past match=w403:i32)  [unwired: 1 in, 3 out]
        n172 = Greater Or Equal To 0?(x=w403) -> (x >= 0?=w402:bool)
        n173 = case shown="True" w402 {
          tunnel: ["Tunnel Speed Settling" ("f") w419] -> w401
          tunnel: w400 -> [_ w423]
          frame False {
          }
          frame True {
            n174 = Greater?(x=w423, y=15) -> (0:w422:bool)
            n175 = Select(t="Modbus Error", s=w422, f="Start") -> (s? t:f=w419:string)
          }
        }
        n176 = call "Set EnFlo Tunnel inlet Fans.vi"("Tunnel Velocity m/s"=w398) -> ("Error Message"=w407:string)
        n177 = Concatenate Strings(w405, w407) -> (w406:string)
      }
      frame "Modbus Error" {
        n178 = disable-structure shown="Enabled" {
          disable-tunnel: [w433 w468] -> w426
          disable-tunnel: "Reset EnFlo Tunnel Modbus" -> [w432 w468]
          frame Disabled {
            n179 = Get Date/Time In Seconds() -> (seconds since 1Jan1904=w439:timestamp)
            n180 = call <vilib>:"LV70TimeStampToDateRec.vi"("time stamp"=w439) -> ("date time rec"=w440:T13)
            n181 = Unbundle By Name(w440) -> ("hour"=w442:i32, "day of week"=w441:i32)
            n182 = In Range and Coerce(upper limit=16 ("lower limit"), x=w442, lower limit=8) -> (In Range?=w444:bool)  [unwired: 1 out]
            n183 = In Range and Coerce(upper limit=7, x=w441, lower limit=1) -> (In Range?=w443:bool)  [unwired: 1 out]
            n184 = And(x=w444, y=w443) -> (x .and. y?=w434:bool)
            n185 = case shown="True" w434 {
              tunnel: [w445 w447] -> w433
              tunnel: w432 -> [w445 w446]
              frame False {
              }
              frame True {
                n186 = stacked-sequence {
                  seq-local: [_ w451 _ _] -> [_ _ w455 _]
                  seq-local: [_ _ w454 _] -> [_ _ _ w463]
                  tunnel: [_ _ _ w461] -> w447
                  tunnel: w446 -> [_ _ _ w462]
                  frame #0 {
                    n187 = call "Email_With_Log.vi"("recipients"=string[] ["paulhayden28@gmail.com", "p.hayden@surrey.ac.uk"], "subject ([No Subject])"="Modbus Error", "message"="Please come and investigate") -> ()  [unwired: 1 in, 3 out]
                  }
                  frame #1 {
                    n188 = call "Wait_Seconds_with_display.vi"("Message"="Press Stop when Ready to make a Decision Regard the Modbus error", "Seconds to wait"=1800 ("y")) -> ("Stopped"=w451:bool)  [unwired: 1 out]
                  }
                  frame #2 {
                    n189 = case shown="True" w455 {
                      tunnel: [FALSE ("T button?") w457] -> w454
                      frame False {
                      }
                      frame True {
                        n190 = Two Button Dialog(message="Do you want to investigate the Modbus error?", 1:"No, Just do the usual Reset" ("F button name (\"Cancel\")"), 2:"Yes" ("T button name (\"OK\")")) -> (T button?=w457:bool)
                      }
                    }
                  }
                  frame #3 {
                    n191 = case shown="True" w463 {
                      tunnel: [w464 "Start"] -> w461
                      tunnel: w462 -> [w464 _]
                      frame False {
                      }
                      frame True {
                        n192 = call "Wait_Seconds_with_display.vi"("Message"="Press Stop when you want the code to try again", "Seconds to wait"=4000.0) -> ()  [unwired: 2 out]
                      }
                    }
                  }
                }
              }
            }
          }
          frame Enabled {
          }
        }
        n193 = Less?(x=w429, y=30) -> (x < y?=w427:bool)
      }
      frame "Reset EnFlo Tunnel Modbus" {
        w470 = "EnFlo_Tunnel:Modbus:Reset"
        n194 = Less?(x=w477, y=30) -> (x < y?=w475:bool)
        n195 = Build Array(w470) -> (w474:string[])
        n196 = stacked-sequence {
          tunnel: w474 -> [w483 _ w488 _]
          frame #0 {
            n197 = Build Array(1.0) -> (w481:dbl[])
            n198 = call "ASYNC_Adam_client.vi"("Values"=w481, "Channel Names"=w483) -> ()  [unwired: 1 in, 2 out]
          }
          frame #1 {
            n199 = call "Wait_Seconds_with_display.vi"("Message"="Resetting EnFlo_Tunnel Modbus", "Seconds to wait"=15.0) -> ()  [unwired: 1 in, 1 out]
          }
          frame #2 {
            n200 = Build Array(0.0) -> (w486:dbl[])
            n201 = call "ASYNC_Adam_client.vi"("Values"=w486, "Channel Names"=w488) -> ()  [unwired: 1 in, 2 out]
          }
          frame #3 {
            n202 = call "Wait_Seconds_with_display.vi"("Message"="Reconnecting EnFlo_Tunnel Modbus", "Seconds to wait"=15.0) -> ()  [unwired: 1 in, 1 out]
          }
        }
        n203 = Bundle By Name(cluster=errorcluster {"status"=FALSE, "code"=0, "source"=""} ("error in (no error)"), "status"=TRUE) -> (w473:errorcluster)
        n204 = call "EnFlo_Error_Handler.vi"("error in (no error)"=w473, "Error Type"=w470, "Dialog Box (F)"=FALSE) -> ()  [unwired: 1 in, 2 out]
      }
      frame "Tunnel Speed Settling" {
        n205 = local read "Settling Time (s)"() -> (w491:dbl)
        n206 = Greater Than 0?(x=w491) -> (x > 0?=w495:bool)
        n207 = Equal?(x=Tunnel_speed_mode."Set Speed then wait" ("Mode"), y=w492) -> (x = y?=w494:bool)
        n208 = Compound Arithmetic op=AND(w494, w495) -> (w496:bool)
        n209 = case shown="True" w496 {
          tunnel: w491 -> [_ w501]
          frame False {
          }
          frame True {
            n210 = call "Wait_Seconds_with_display.vi"("Message"="Tunnel speed settling", "Seconds to wait"=w501) -> ()  [unwired: 2 out]
          }
        }
      }
      frame "Do Not Link To Server" {
        # "Clamped"
        # "Pre vel"
        # "Tweak"
        # "Tweaked\nVel"
        # "Volts"
        n211 = stacked-sequence {
          seq-local: [w516 _ _ _ _ _ _] -> [_ w531 w537 w546 w562 w621 _]
          seq-local: [_ _ w532 _ _ _ _] -> [_ _ _ _ w566 _ _]
          seq-local: [_ _ _ w542 _ _ _] -> [_ _ _ _ w561 _ w636]
          seq-local: [_ _ _ w545 _ _ _] -> [_ _ _ _ w564 w616 _]
          seq-local: [_ _ _ _ w563 _ _] -> [_ _ _ _ _ w615 _]
          seq-local: [_ _ _ w547 _ _ _] -> [_ _ _ _ _ _ w642]
          seq-local: [w513 _ _ _ _ _ _] -> [_ _ _ _ _ _ w626]
          seq-local: [_ w522 _ _ _ _ _] -> [_ _ _ w540 _ _ w641]
          tunnel: w506 -> [_ w523 _ _ _ _ _]
          tunnel: w504 -> [w517 _ _ w554 _ _ w638]
          tunnel: w507 -> [_ _ _ _ w565 w610 _]
          tunnel: [_ w521 _ _ _ _ _] -> w505
          tunnel: w503 -> [_ w520 _ _ _ _ _]
          frame #0 {
            n212 = Concatenate Strings(w517, "_Calib" ("Substring"), ".xls" ("string")) -> (w511:string)
            n213 = call "Setup_Filepath.vi"("Setup File Type"=Setup_Filetype."Speed Calib Tweaks", "Filename in"=w511) -> ("Filename Out"=w510:path)  [unwired: 1 out]
            n214 = call "Setup_Filepath.vi"("Setup File Type"=Setup_Filetype."Speed Calib Tweaks", "Filename in"="Current_Values.xls" ("name or relative path")) -> ("Filename Out"=w513:path)  [unwired: 1 out]
            n215 = call "Read_File_No_Error.vi"("Filename"=w510) -> ("string"=w516:string)  [unwired: 2 in, 7 out]
          }
          frame #1 {
            w525 = -2.0  # Min
            n216 = call "Get_value_from_string.vi"("Input string"=w531, "Variable name"="Maximum_Allowable_Tunnel_Speed") -> ("Value"=w524:dbl)  [unwired: 1 in, 1 out]
            n217 = In Range and Coerce(upper limit=w524, x=w523, lower limit=w525) -> (coerced(x)=w522:dbl)  [unwired: 1 out]
            n218 = Greater?(x=w523, y=w524) -> (0:w526:bool)
            n219 = Format Into String(format string="Req Speed Dem = %.1f m/s, Max allowable = %.1f m/s", initial string=w520, w523, w524) -> (resulting string=w528:string)  [unwired: 1 in, 1 out]
            n220 = Select(t=w528, s=w526, f="") -> (s? t:f=w521:string)
          }
          frame #2 {
            n221 = call "Get_Characters_from_string.vi"("Input string"=w537, "Variable name"="VI_to_Remote_Call") -> ("Value"=w535:string)  [unwired: 1 in, 1 out]
            n222 = global read "Constants_global.vi" "EnFlo SW Folder"() -> (w533:path)
            n223 = call "String_to_Pathname.vi"("Input String"=w535) -> ("path"=w536:path)
            n224 = Path to Array of Strings(0:w536) -> (2:w534:string[])  [unwired: 1 out]
            n225 = call "Build_Pathname.vi"("PathElements"=w534, "PathnameIn"=w533) -> ("AppendedPath"=w532:path)
          }
          frame #3 {
            n226 = local write "Tunnel Velocity m/s"(w540) -> ()
            n227 = call "Add_to_speed_calib_file.vi"("Desired Velocity"=w540, "Max Velocity"=0.0, "Rig Name"=w554, "Mode"=enum16{"Add Row", "Get Error Value"}."Get Error Value") -> ("Tweaked Demand"=w545:dbl, "Calib Tweak %"=w547:dbl)  [unwired: 2 in]
            n228 = Less?(x=w545, y=0.01) -> (x < y?=w543:bool)
            n229 = call "Get_value_from_string.vi"("Input string"=w546, "Variable name"="Calibration_Coefficient_Offset_C") -> ("Value"=w548:dbl)  [unwired: 1 in, 1 out]
            n230 = call "Get_value_from_string.vi"("Input string"=w546, "Variable name"="Calibration_Coefficient_Slope_M") -> ("Value"=w550:dbl)  [unwired: 1 in, 1 out]
            n231 = Multiply(x=w550, y=w545) -> (x*y=w549:dbl)
            n232 = Add(x=w548, y=w549) -> (x+y=w541:dbl)
            n233 = case shown="False" w543 {
              tunnel: w546 -> [_ w557]
              tunnel: [w555 w556] -> w542
              tunnel: w541 -> [w555 _]
              frame False {
              }
              frame True {
                n234 = call "Get_value_from_string.vi"("Input string"=w557, "Variable name"="Zero_Velocity_Output_Voltage") -> ("Value"=w556:dbl)  [unwired: 1 in, 1 out]
              }
            }
          }
          frame #4 {
            w560 = TRUE  # Dialog Box
            n235 = while {
              tunnel: w566 -> [w576]
              tunnel: w565 -> [w575]
              tunnel: w564 -> [w574]
              tunnel: [w573] -> w563
              shift-right: [w571] -> _
              shift-left: _ -> [w570]
              tunnel: [w569] -> w559
              tunnel: w562 -> [w568]
              tunnel: w561 -> [w567]
              stop <- TRUE stop-if-true
              n236 = case shown="\"Is tunnel speed allowable?\"" w575 {
                tunnel: w576 -> [_ w596]
                tunnel: w574 -> [_ w583]
                tunnel: [w578 w585] -> w573
                tunnel: [w578 w583] -> w571
                tunnel: w570 -> [w578 w584]
                tunnel: [errorcluster {"status"=FALSE, "code"=0, "source"=""} ("error out") w579] -> w569
                tunnel: w568 -> [_ _]
                tunnel: w567 -> [_ w582]
                frame "Is tunnel speed allowable?" {
                }
                frame "Set Speed then wait", Default {
                  n237 = Open VI Reference(type specifier VI Refnum (for type only)=refnum<vi> refnum, vi path=w596) -> (vi reference=w594:refnum<vi>, error out=w593:errorcluster)  [unwired: 1 in, 3 out]
                  n238 = property class="VI Interface Type 1"(reference=w594, error in=w593) -> (reference out=w591:refnum<vi>, error out=w592:errorcluster, "Front Panel.Open"=w590:bool)
                  n239 = case shown="False" w590 {
                    tunnel: w592 -> [w601 w604]
                    tunnel: w591 -> [w600 w605]
                    tunnel: [w599 w605] -> w589
                    tunnel: [w598 w604] -> w588
                    tunnel: [0.0 ("Tweaked Demand") w603] -> w585
                    tunnel: w584 -> [_ w603]
                    frame False {
                      n240 = property class="VI Interface Type 1"(reference=w600, error in=w601, "Front Panel.Open"=TRUE ("Front Panel Window:Open")) -> (reference out=w599:refnum<vi>, error out=w598:errorcluster)
                    }
                    frame True {
                    }
                  }
                  n241 = call-by-ref "?"(reference=w589, error in=w588, "Demand"=w582) -> (reference out=w586:refnum<vi>, error out=w587:errorcluster, "error out"=w580:errorcluster)
                  n242 = Close Reference(reference=w586, error in (no error)=w587) -> (error out=w581:errorcluster)
                  n243 = Select(t=w581, s=w581, f=w580) -> (s? t:f=w579:errorcluster)
                }
              }
            }
            n244 = call "EnFlo_Error_Handler.vi"("error in (no error)"=w559, "Dialog Box (F)"=w560) -> ()  [unwired: 1 in, 3 out]
          }
          frame #5 {
            n245 = Subtract(x=w615, y=w616) -> (x-y=w614:dbl)
            n246 = Absolute Value(x=w614) -> (abs(x)=w608:dbl)
            n247 = call "Get_value_from_string.vi"("Input string"=w621, "Variable name"="Settling_time_Offset_C") -> ("Value"=w617:dbl)  [unwired: 1 in, 1 out]
            n248 = call "Get_value_from_string.vi"("Input string"=w621, "Variable name"="Settling_time_Slope_M") -> ("Value"=w619:dbl)  [unwired: 1 in, 1 out]
            n249 = Multiply(x=w619, y=w608) -> (x*y=w618:dbl)
            n250 = Add(x=w617, y=w618) -> (x+y=w609:dbl)
            n251 = Greater?(x=w608, y=0.05) -> (0:w606:bool)
            n252 = Equal?(x=Tunnel_speed_mode."Set Speed then wait" ("Mode"), y=w610) -> (x = y?=w612:bool)
            n253 = Compound Arithmetic op=AND(w606, w612) -> (w611:bool)
            n254 = case shown="False" w611 {
              tunnel: w609 -> [_ w623]
              frame False {
              }
              frame True {
                n255 = call "Wait_Seconds_with_display.vi"("Message"="Tunnel speed settling", "Seconds to wait"=w623) -> ()  [unwired: 2 out]
              }
            }
          }
          frame #6 {
            n256 = Concatenate Strings(w638, ":Speed:Dem_Voltage" ("string")) -> (w633:string)
            n257 = Bundle By Name(cluster=T7 {"Ch Name"="", "Type"="", "Function"=enum."Analogue Input", "Ch State"=enum."On", "Calibration type"="", "A"=0.0, "B"=0.0, "C"=0.0, "D"=0.0, "Comments"="", "Address"={"Main"=0, "Ch."=0, "Sub"=0, "Port Name"=""}, "String"="", "Duty"=0} ("Ch Discription"), "Ch Name"=w633, "Type"=T6 "Hold Value", "Calibration type"=T5 "", "Ch State"=Channel_State."On") -> (w627:T7)
            n258 = Bundle By Name(cluster=T11 {"Channel Name"="", "New Value"=0.0, "!Auto_Off"=FALSE} ("Update Scan Value Cluster"), "Channel Name"=w633, "New Value"=w636) -> (w639:T11)
            n259 = call "Value_to_string.vi"("Value"=w642, "Label for value"="Calib Tweak") -> ("Output string"=w644:string)  [unwired: 1 in]
            n260 = call "Value_to_string.vi"("Value"=w641, "Label for value"="Velocity Demand") -> ("Output string"=w643:string)  [unwired: 1 in]
            n261 = Concatenate Strings(w644, w643) -> (w625:string)
            n262 = Build Array(w627) -> (w628:T7[])
            n263 = Build Array(w639) -> (w629:T11[])
            n264 = call "Write Characters with check.vi"("String to Write"=w625, "file (use dialog)"=w626) -> ()  [unwired: 2 in, 1 out]
            n265 = call "Read_Write_Local_table.vi"("Mode"=Global_mode."Write Global to File", "Ch Values in"=w629, "Channels Descriptions In"=w628) -> ()  [unwired: 3 out]
          }
        }
      }
    }
  }
  "Error String" <- w10
